vi "TimeShiftDataI8.vi"(3 "output cluster":T1, 4 "Array In":i8[][](array[numeric])) -> (0 "Array Out":i8[][](array[numeric]), 1 "x-y":u32)   [LabVIEW 2022 SP3]
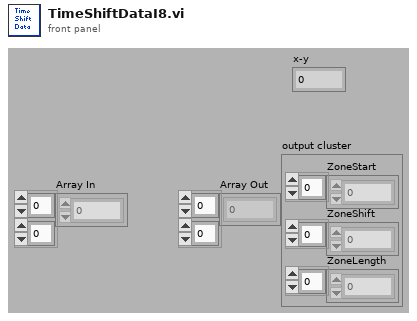
[diagram p1: front panel]
types:
  T1 = cluster{"ZoneStart":sgl[], "ZoneShift":sgl[], "ZoneLength":sgl[]}
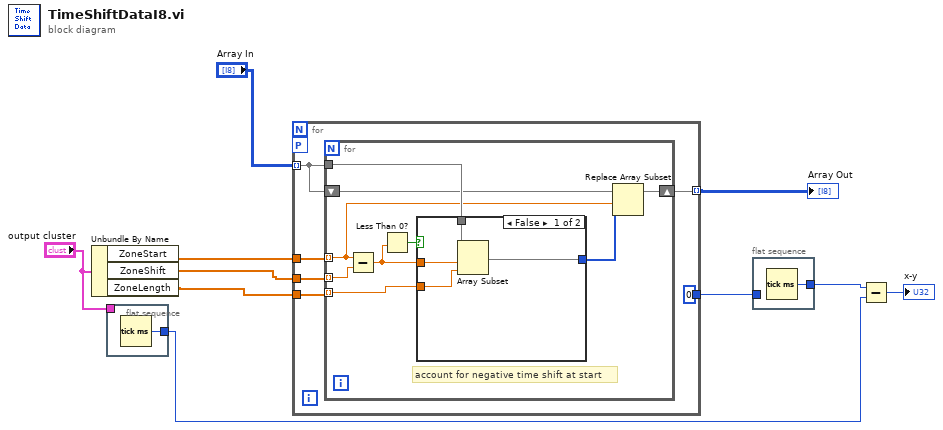
[diagram p0: block diagram]
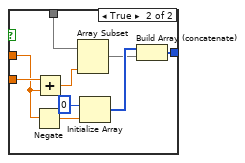
[diagram p2: hidden frame]
diagram:
  n1 = Unbundle By Name("output cluster") -> ("ZoneStart"=w8:sgl[], "ZoneShift"=w7:sgl[], "ZoneLength"=w6:sgl[])
  n2 = flat-sequence {
    tunnel: [w11] -> w2
    tunnel: "output cluster" -> [_]
    frame #0 {
      n3 = Tick Count (ms)() -> (millisecond timer value=w11:u32)
    }
  }
  n4 = for {
    tunnel: "Array In" -> [w13] mode=indexing
    tunnel: w8 -> [w17]
    tunnel: w7 -> [w16]
    tunnel: w6 -> [w15]
    workers-P: _ -> [_]
    tunnel: [w14] -> w9 mode=indexing
    tunnel: [0] -> w5
    n5 = for {
      tunnel: w17 -> [w19] mode=indexing
      tunnel: w15 -> [w26] mode=indexing
      tunnel: w16 -> [w25] mode=indexing
      tunnel: w13 -> [w22]
      shift-right: [w21] -> w14
      shift-left: w13 -> [w20]
      # "account for negative time shift at start"
      n6 = Subtract(x=w19, y=w25) -> (x-y=w23:sgl)
      n7 = Less Than 0?(x=w23) -> (x < 0?=w24:bool)
      n8 = case shown="False" w24 {
        tunnel: w22 -> [w30 w38]
        tunnel: w26 -> [w28 w39]
        tunnel: [w29 w33] -> w18
        tunnel: w23 -> [w27 w36]
        frame False {
          n9 = Array Subset(array=w30, index=w27, length=w28) -> (w29:i8[])
        }
        frame True {
          n10 = Negate(x=w36) -> (-x=w31:sgl)
          n11 = Add(x=w39, y=w36) -> (x+y=w32:sgl)
          n12 = Array Subset(array=w38, length=w32) -> (w34:i8[])  [unwired: 1 in]
          n13 = Initialize Array(i16 0, w31) -> (w35:i16[])
          n14 = Build Array (concatenate)(w35, w34) -> (w33:i16[])
        }
      }
      n15 = Replace Array Subset(array=w20, new element=w18, index=w19) -> (w21:i8[])
    }
  }
  "Array Out" <- w9
  n16 = flat-sequence {
    tunnel: [w40] -> w3
    tunnel: w5 -> [_]
    frame #0 {
      n17 = Tick Count (ms)() -> (millisecond timer value=w40:u32)
    }
  }
  n18 = Subtract(x=w3, y=w2) -> (x-y=→"x-y":u32)
